vi "ActiveX - WordTables2StringArray.vi"(8 "Error In":errorcluster, 11 "File Path Control":path) -> (0 "Error Out":errorcluster, 1 "column":i32, 2 "row":i32, 3 "Array":string[][](array[string]))   [LabVIEW 2019]
doc: "Word中表格读取为LabVIEW数组\n\nApplication 属性 (Word) 代表 Microsoft Word 应用程序。\nApplication.Documents 代表所有打开的文档。\n\nDocuments对象 open方法 可以打开一个word文档。\n 需要的最简单的参数是文件名。\n\nTables对象 是Table对象的一个集合。\n 属性：Count，表示集合中的表的数目。\n 方法：Item，获取Tables集合中的一个Table对象。\n 需要参数是index，用来索引的。\n\nTable对象 表示单个表格\n 属性：Columns \n 属性：Rows \n 方法：Cell\n 参数：Row\n 参数：Column\n\nColumns 是 Column 的集合对象\nRows 是 Row 的集合对象\n 属性：Count 代表集合中的行数和列数\n\nCell 对象 代表表格中的一个单元格。\n\nRange 对象 代表指定对象所含的部分文档。\n表示文档中的一个连续区域。 每个 Range 对象由一个起始字符位置和一个终止字符位置定义。\n 属性：Text 返回该区域的无格式纯文本。"
panel:
  # "Application 属性 (Word) 代表 Microsoft Word 应用程序。\nApplication.Documents 代表所有打开的文档。\n\nDocuments对象 open方法 可以打开一个word文档。\n\t需要的最简单的参数是文件名。\n\nTables对象 是Table对象的一个集合。\n\t属性：Count，表示集合中的表的数目。\n\t方法：Item，获取Tables集合中的一个Table对象。\n\t\t需要参数是index，用来索引的。\n\nTable对象 表示单个表格\n\t属性：Columns \n\t属性：Rows \n\t方法：Cell\n\t\t参数：Row\n\t\t参数：Column\n\nColumns 是 Column 的集合对象\nRows 是 Row 的集合对象\n\t属性：Count 代表集合中的行数和列数\n\nCell 对象 代表表格中的一个单元格。\n\nRange 对象 代表指定对象所含的部分文档。\n表示文档中的一个连续区域。 每个 Range 对象由一个起始字符位置和一个终止字符位置定义。\n\t属性：Text 返回该区域的无格式纯文本。"
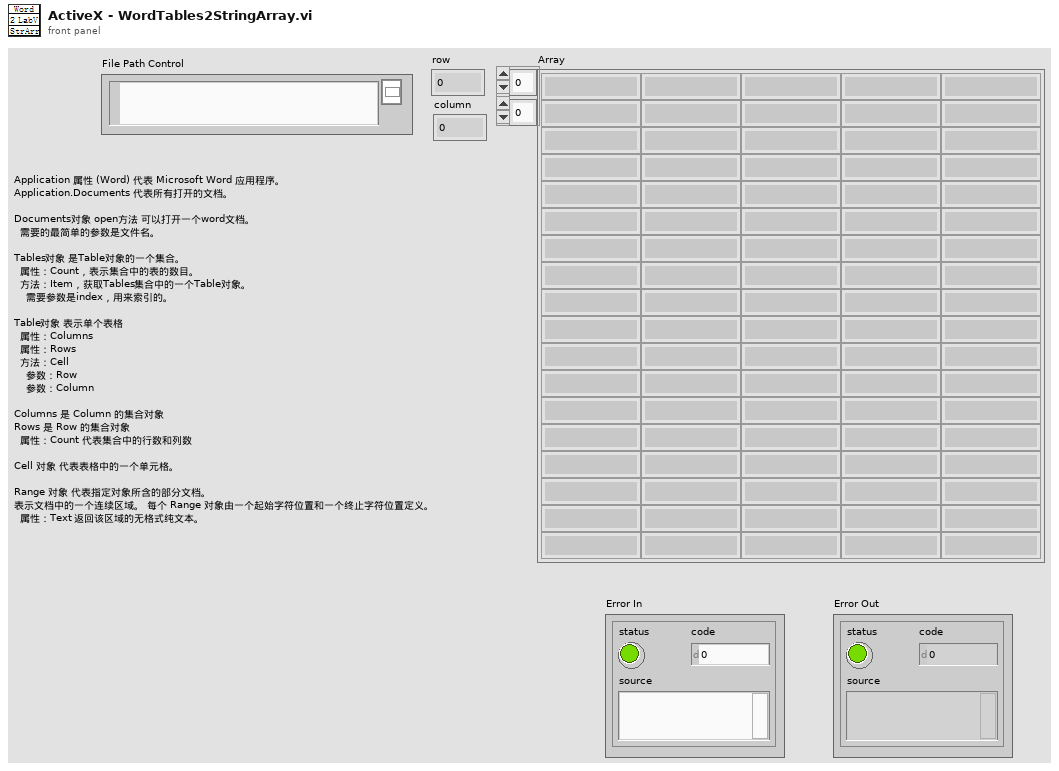
[diagram p1: front panel]
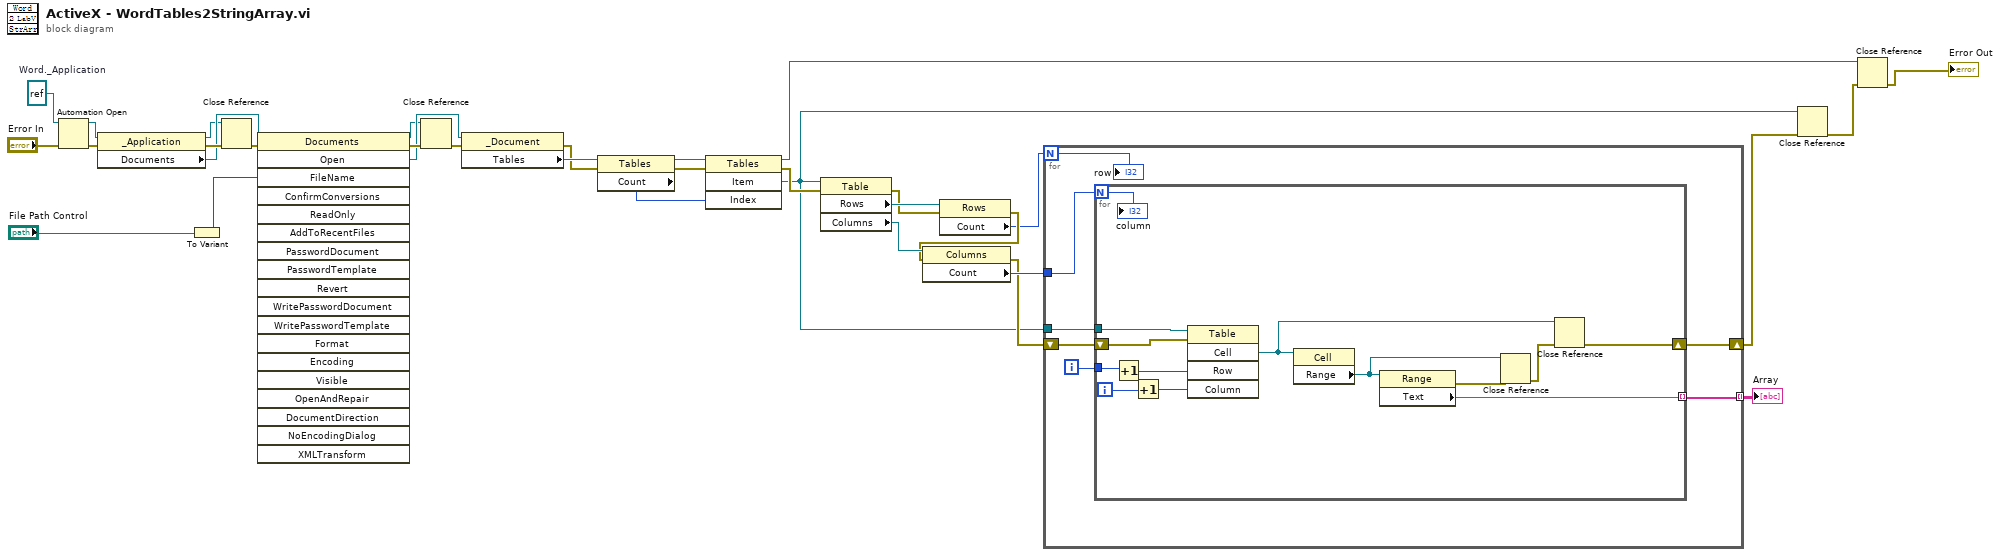
[diagram p0: block diagram]
diagram:
  w33 = refnum<k7> refnum  # Word._Application
  n1 = Automation Open(error in (no error)="Error In", Automation Refnum=w33) -> (Automation Refnum=w32:refnum<k7>, error out=w31:errorcluster)  [unwired: 2 in]
  n2 = property class="_Application"(reference=w32, error in=w31) -> (reference out=w22:refnum<k7>, error out=w30:errorcluster, "Documents"=w29:refnum<k7>)
  n3 = To Variant(anything="File Path Control") -> (Variant=w28:variant)
  n4 = Close Reference(reference=w22, error in (no error)=w30) -> (error out=w23:errorcluster)
  n5 = invoke class="Documents" method="Open"(reference=w29, error in=w23, "FileName"=w28) -> (reference out=w24:refnum<k7>, error out=w27:errorcluster, "Open"=w26:refnum<k7>)  [unwired: 16 in, 16 out]
  n6 = Close Reference(reference=w24, error in (no error)=w27) -> (error out=w25:errorcluster)
  n7 = property class="_Document"(reference=w26, error in=w25) -> (error out=w18:errorcluster, "Tables"=w19:refnum<k7>)  [unwired: 1 out]
  n8 = property class="Tables"(reference=w19, error in=w18) -> (reference out=w17:refnum<k7>, error out=w16:errorcluster, "Count"=w15:i32)
  n9 = invoke class="Tables" method="Item"(reference=w17, error in=w16, "Index"=w15) -> (reference out=w2:refnum<k7>, error out=w12:errorcluster, "Item"=w3:refnum<k7>)  [unwired: 1 in, 1 out]
  n10 = property class="Table"(reference=w3, error in=w12) -> (error out=w11:errorcluster, "Rows"=w14:refnum<k7>, "Columns"=w13:refnum<k7>)  [unwired: 1 out]
  n11 = property class="Rows"(reference=w14, error in=w11) -> (error out=w10:errorcluster, "Count"=w9:i32)  [unwired: 1 out]
  n12 = property class="Columns"(reference=w13, error in=w10) -> (error out=w7:errorcluster, "Count"=w8:i32)  [unwired: 1 out]
  n13 = for {
    N: w9 -> [w34]
    tunnel: w8 -> [w40]
    tunnel: w3 -> [w39]
    tunnel: [w36] -> w1 mode=indexing
    shift-right: [w35] -> w4
    shift-left: w7 -> [w37]
    i -> [w38]
    n14 = for {
      N: w40 -> [w42]
      tunnel: w39 -> [w53]
      tunnel: w38 -> [w49]
      tunnel: [w41] -> w36 mode=indexing
      shift-right: [w43] -> w35
      shift-left: w37 -> [w48]
      i -> [w50]
      n15 = Increment(x=w49) -> (x+1=w52:i32)
      n16 = Increment(x=w50) -> (x+1=w51:i32)
      n17 = invoke class="Table" method="Cell"(reference=w53, error in=w48, "Row"=w52, "Column"=w51) -> ("Cell"=w44:refnum<k7>)  [unwired: 1 in, 4 out]
      n18 = property class="Cell"(reference=w44) -> ("Range"=w47:refnum<k7>)  [unwired: 1 in, 2 out]
      n19 = property class="Range"(reference=w47) -> (error out=w46:errorcluster, "Text"=w41:string)  [unwired: 1 in, 1 out]
      n20 = Close Reference(reference=w47, error in (no error)=w46) -> (error out=w45:errorcluster)
      n21 = Close Reference(reference=w44, error in (no error)=w45) -> (error out=w43:errorcluster)
      "column" <- w42
    }
    "row" <- w34
  }
  "Array" <- w1
  n22 = Close Reference(reference=w3, error in (no error)=w4) -> (error out=w5:errorcluster)
  n23 = Close Reference(reference=w2, error in (no error)=w5) -> (error out=→"Error Out":errorcluster)
